vi "Get Exposure Time.vi"(8 "error in (no error)":errorcluster, 11 "Camera in":refnum<class "Camera.lvclass">) -> (0 "error out":errorcluster, 2 "Time (us)":dbl, 3 "Camera":refnum<class "Camera.lvclass">)   [LabVIEW 2020, in "Camera.lvclass"]
uses:
  Camera.lvclass
  Camera.lvclass/Camera.ctl
  Check Not Disconnected.vi
  <vilib>/Utility/error.llb/Error Cluster From Error Code.vi
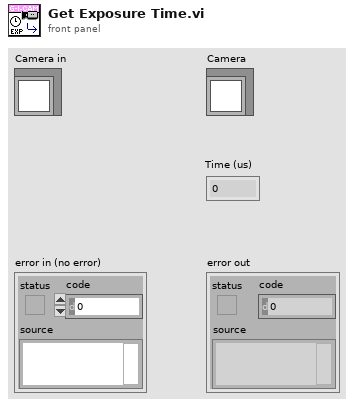
[diagram p1: front panel]
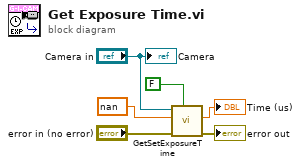
[diagram p0: block diagram]
diagram:
  n1 = call "GetSetExposureTime.vi"("Set?"=FALSE, "error in (no error)"="error in (no error)", "Value In"=nan, "Camera in"="Camera in") -> ("error out"=→"error out":errorcluster, "Value Out"=→"Time (us)":dbl)  [unwired: 6 in]
  "Camera" <- "Camera in"
